vi "Set Report Font.vi"(4 "text color (unchanged)":u32(colorbox)=16777216, 5 "error in (no error)":errorcluster, 6 "font settings":T3={"charset (-1)"=-1, "weight (-1)"=-1, "name"="", "size"=" "}, 7 "text options":T2, 8 "report in":T1) -> (0 "error out":errorcluster, 3 "report out":T1)   [LabVIEW 2015]
doc: "Sets the font properties of the report, including those in the headers and footers."
uses:
  <vilib>/Utility/NIReport.llb/Generate Report Object Reference.ctl
  <vilib>/Utility/NIReport.llb/NI_report.lvclass
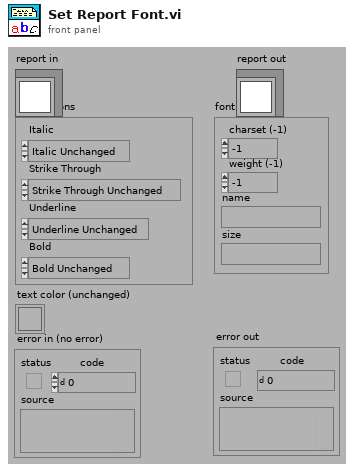
[diagram p1: front panel]
types:
  T1 = typedef "Generate Report Object Reference.ctl" = refnum<class "NI_report.lvclass">
  T2 = cluster{"Italic":enum16{"Italic Unchanged", "Italic On", "Italic Off"}, "Strike Through":enum16{"Strike Through Unchanged", "Strike Through On", "Strike Through Off"}, "Underline":enum16{"Underline Unchanged", "Underline On", "Underline Off"}, "Bold":enum16{"Bold Unchanged", "Bold On", "Bold Off"}}
  T3 = cluster{"charset (-1)":i16, "weight (-1)":i16, "name":string, "size":string}
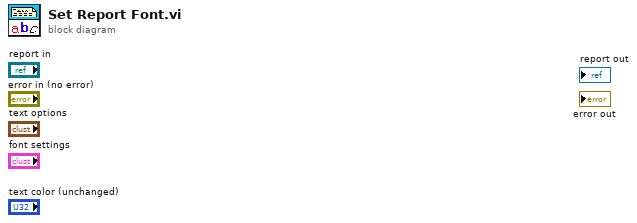
[diagram p0: block diagram]
diagram:
